vi "shutdown.vi"() -> ()   [LabVIEW 2015]
uses:
  Windows/System32/user32.dll
panel:
  in  "stop":bool
  out "error out":errorcluster
  in  "error in (no error)":errorcluster
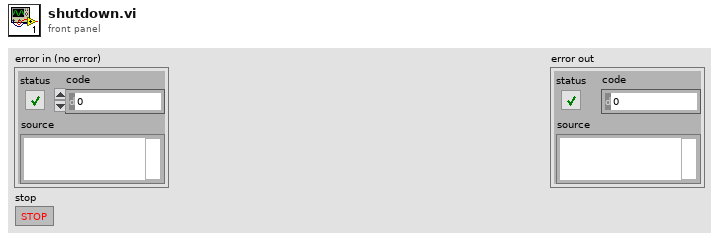
[diagram p1: front panel]
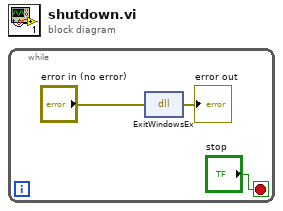
[diagram p0: block diagram]
diagram:
  n1 = while {
    stop <- "stop" stop-if-true
    n2 = dll-call lib="C:/Windows/System32/user32.dll" fn="ExitWindowsEx"(error in="error in (no error)") -> (error out=→"error out":errorcluster)  [unwired: 3 in, 1 out]
  }
